vi "BuildRoomFilter.vi"(4 "BedVacant":bool, 5 "RoomNumFlags":T1={"Flag State"=[1, 3, 5, 7]}, 6 "InputCondition":string, 7 "Filter":T2, 8 "error in":errorcluster, 9 "Filter Text":string, 10 "To":timestamp, 11 "From":timestamp) -> (0 "error out":errorcluster, 2 "condition":string)   [LabVIEW 2015, in "DatabaseApi.lvlib"]
uses:
  DatabaseApi.lvlib
  TypeDef/Room/RoomTableFilterRing.ctl
  LVClasses/Flags/ColorFlags.ctl
  TypeDef/Room/RoomTableDbTableName.ctl
  <vilib>/addons/database/Connection.llb/DB Tools Open Connec (String).vi
  <vilib>/addons/database/Auxilliary.llb/DB Tools Format Datetime String (Time Stamp).vi
  <vilib>/addons/database/NI_Database_API.lvlib
  LVClasses/Flags/Flags.lvclass
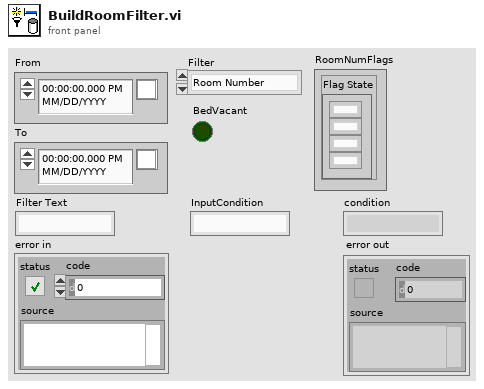
[diagram p1: front panel]
types:
  T1 = typedef "Flags.lvclass/ColorFlags.ctl" = cluster{"Flag State":u8[]}
  T2 = typedef "DatabaseApi.lvlib/RoomTableFilterRing.ctl" = enum16{"Room Number", "Event Time", "Flags", "Bed Vacant", "In Room Personnel"}
  T3 = typedef "DatabaseApi.lvlib/RoomTableDbTableName.ctl" = string
  T4 = typedef "NI_Database_API.lvlib/Conn ObjectReference.ctl" = refnum<k1>
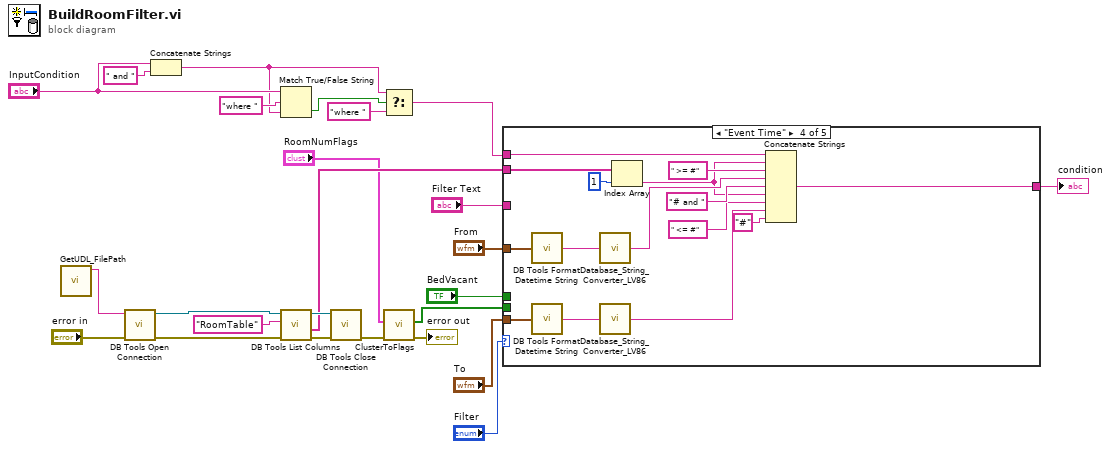
[diagram p0: block diagram]
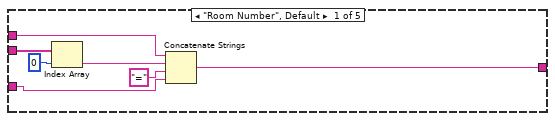
[diagram p2: hidden frame]
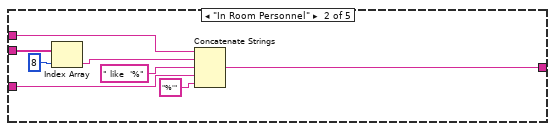
[diagram p3: hidden frame]
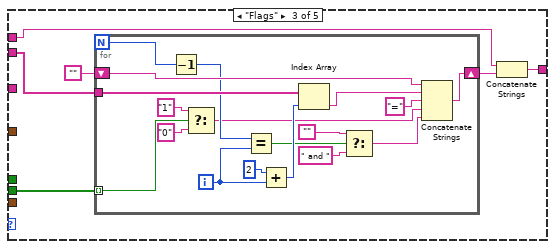
[diagram p4: hidden frame]
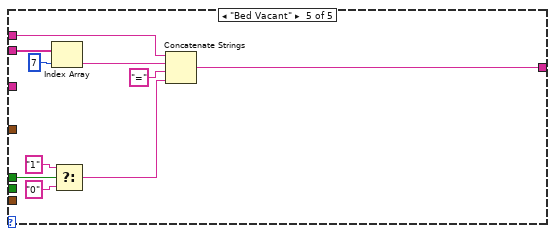
[diagram p5: hidden frame]
diagram:
  n1 = call "GetUDL_FilePath.vi"() -> ("UDL file path"=w23:string)  [unwired: 11 in]
  n2 = call-poly <vilib>:"DB Tools Open Connection.vi"("error in (no error)"="error in", "connection information"=w23) -> ("error out"=w22:errorcluster, "connection reference"=w20:T4)  [unwired: 6 in]
  n3 = Concatenate Strings("InputCondition", " and " ("string")) -> (w9:string)
  n4 = Match True/False String(2:w9, 3:"where " ("string"), 4:"InputCondition") -> (0:w12:bool)  [unwired: 1 out]
  n5 = call <vilib>:"DB Tools List Columns.vi"("error in (no error)"=w22, "table"=T3 "RoomTable" ("RoomTableName"), "connection reference"=w20) -> ("error out"=w19:errorcluster, "columns"=w7:string[], "connection reference out"=w18:T4)  [unwired: 1 in, 1 out]
  n6 = call <vilib>:"DB Tools Close Connection.vi"("error in (no error)"=w19, "connection reference"=w18) -> ("error out"=w4:errorcluster)  [unwired: 5 in]
  n7 = Select(t=w9, s=w12, f="where " ("string")) -> (s? t:f=w11:string)
  n8 = call "ClusterToFlags.vi"("error in"=w4, "RoomNumFlags"="RoomNumFlags") -> ("error out"=→"error out":errorcluster, "State"=w2:bool[])  [unwired: 8 in]
  n9 = case shown="\"Event Time\"" "Filter" {
    tunnel: "To" -> [_ _ _ w79 _]
    tunnel: "From" -> [_ _ _ w78 _]
    tunnel: [w30 w38 w46 w75 w88] -> w16
    tunnel: "Filter Text" -> [w32 w40 _ _ _]
    tunnel: w11 -> [w29 w37 w41 w68 w87]
    tunnel: w7 -> [w27 w35 w44 w65 w85]
    tunnel: "BedVacant" -> [_ _ _ _ w80]
    tunnel: w2 -> [_ _ w45 _ _]
    frame "Room Number", Default {
      n10 = Index Array(array=w27, index=0) -> (element=w26:string)
      n11 = Concatenate Strings(w29, w26, "=" ("string"), w32) -> (w30:string)
    }
    frame "In Room Personnel" {
      n12 = Index Array(array=w35, index=8) -> (element=w34:string)
      n13 = Concatenate Strings(w37, w34, " like  '%" ("string"), w40, "%'" ("string")) -> (w38:string)
    }
    frame "Flags" {
      n14 = for {
        N -> [w54]
        tunnel: w45 -> [w55] mode=indexing
        tunnel: w44 -> [w62]
        shift-right: [w61] -> w42
        shift-left: "" -> [w60]
        i -> [w52]
        n15 = Decrement(x=w54) -> (x-1=w53:i32)
        n16 = Select(t="1" ("string"), s=w55, f="0" ("string")) -> (s? t:f=w51:string)
        n17 = Equal?(x=w53, y=w52) -> (x = y?=w47:bool)
        n18 = Add(x=2 ("index"), y=w52) -> (x+y=w64:i32)
        n19 = Index Array(array=w62, index=w64) -> (element=w59:string)
        n20 = Select(t="", s=w47, f=" and " ("string")) -> (s? t:f=w49:string)
        n21 = Concatenate Strings(w60, w59, "=" ("string"), w51, w49) -> (w61:string)
      }
      n22 = Concatenate Strings(w41, w42) -> (w46:string)
    }
    frame "Event Time" {
      n23 = call-poly <vilib>:"DB Tools Format Datetime String.vi"("time stamp"=w78) -> ("date/time string"=w77:string)
      n24 = call-poly <vilib>:"DB Tools Format Datetime String.vi"("time stamp"=w79) -> ("date/time string"=w73:string)
      n25 = call "Database_String_Converter_LV86.vi"("String Input (date/timeyyyy-mm-dd hh:mm:ss)"=w77) -> ("String Output (mm/dd/yyyy hh:mm:ss AM/PM)"=w72:string)  [unwired: 4 in]
      n26 = call "Database_String_Converter_LV86.vi"("String Input (date/timeyyyy-mm-dd hh:mm:ss)"=w73) -> ("String Output (mm/dd/yyyy hh:mm:ss AM/PM)"=w71:string)  [unwired: 4 in]
      n27 = Index Array(array=w65, index=1) -> (element=w66:string)
      n28 = Concatenate Strings(w68, w66, " >= #" ("string"), w72, "# and " ("string"), w66, " <= #" ("string"), w71, "#" ("string")) -> (w75:string)
    }
    frame "Bed Vacant" {
      n29 = Index Array(array=w85, index=7) -> (element=w86:string)
      n30 = Select(t="1" ("string"), s=w80, f="0" ("string")) -> (s? t:f=w83:string)
      n31 = Concatenate Strings(w87, w86, "=" ("string"), w83) -> (w88:string)
    }
  }
  "condition" <- w16
